vi "Colores_b.vi"() -> ()   [LabVIEW 2017]
panel:
  out "Azul":u32[](array[colorbox])
  out "Verde":u32[](array[colorbox])
  out "Rojo":u32[](array[colorbox])
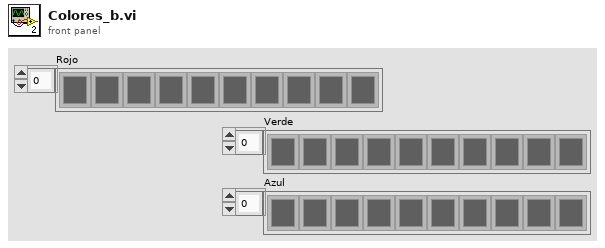
[diagram p1: front panel]
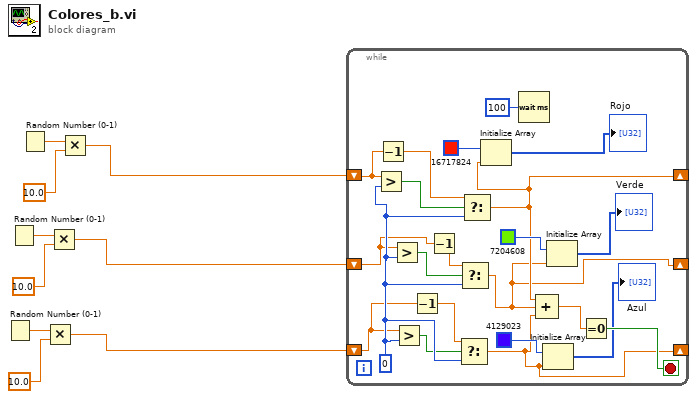
[diagram p0: block diagram]
diagram:
  n1 = Random Number (0-1)() -> (number: 0 to 1=w5:dbl)
  n2 = Random Number (0-1)() -> (number: 0 to 1=w7:dbl)
  n3 = Random Number (0-1)() -> (number: 0 to 1=w9:dbl)
  n4 = Multiply(x=w5, y=10.0) -> (x*y=w1:dbl)
  n5 = Multiply(x=w7, y=10.0) -> (x*y=w2:dbl)
  n6 = Multiply(x=w9, y=10.0) -> (x*y=w3:dbl)
  n7 = while {
    shift-right: [w11] -> _
    shift-left: w2 -> [w24]
    shift-right: [w10] -> _
    shift-left: w1 -> [w22]
    shift-right: [w12] -> _
    shift-left: w3 -> [w27]
    stop <- w19 stop-if-true
    w30 = 0
    n8 = Greater?(x=w27, y=w30) -> (0:w28:bool)
    n9 = Decrement(x=w27) -> (x-1=w26:dbl)
    n10 = Greater?(x=w24, y=w30) -> (0:w29:bool)
    n11 = Greater?(x=w22, y=w30) -> (0:w21:bool)
    n12 = Decrement(x=w22) -> (x-1=w23:dbl)
    n13 = Decrement(x=w24) -> (x-1=w25:dbl)
    n14 = Select(t=w23, s=w21, f=w30) -> (s? t:f=w10:dbl)
    n15 = Select(t=w25, s=w29, f=w30) -> (s? t:f=w11:dbl)
    n16 = Select(t=w26, s=w28, f=w30) -> (s? t:f=w12:dbl)
    n17 = Initialize Array "Initialize Array"(u32 16717824, w12) -> (→"Rojo":u32[])
    n18 = Wait (ms)(milliseconds to wait=u32 100) -> ()  [unwired: 1 out]
    n19 = Compound Arithmetic op=ADD(w12, w11, w10) -> (w20:dbl)
    n20 = Initialize Array "Initialize Array"(u32 4129023, w10) -> (→"Azul":u32[])
    n21 = Initialize Array "Initialize Array"(u32 7204608, w11) -> (→"Verde":u32[])
    n22 = Equal To 0?(x=w20) -> (x = 0?=w19:bool)
  }
